vi "Weather Parse Test.vi"() -> ()   [LabVIEW 2020, in "CDM-Config.lvlib"] (continued)
                 ],\n                    \"WMOidentifier\": [\n                        \"FZAK51 PAFC 021149\"\n                    ],\n                    \"NWSheadline\": [\n                        \"SMALL CRAFT ADVISORY THROUGH WEDNESDAY\"\n                    ],\n                    \"BLOCKCHANNEL\": [\n                        \"EAS\",\n                        \"NWEM\",\n                        \"CMAS\"\n                    ],\n                    \"VTEC\": [\n                        \"/O.NEW.PAFC.SC.Y.9557.251202T1100Z-251204T0200Z/\"\n                    ],\n                    \"eventEndingTime\": [\n                        \"2025-12-03T17:00:00-09:00\"\n                    ]\n                },\n                \"scope\": \"Public\",\n                \"code\": \"IPAWSv1.0\",\n                \"language\": \"en-US\",\n                \"web\": \"http://www.weather.gov\",\n                \"eventCode\": {\n                    \"SAME\": [\n                        \"NWS\"\n                    ],\n                    \"NationalWeatherService\": [\n                        \"SCY\"\n                    ]\n                }\n            }\n        },\n        {\n            \"id\": \"https://api.weather.gov/alerts/urn:oid:2.49.0.1.840.0.7a1ebf60c096e67f68143934abaf6f7cf8a57038.003.1\",\n            \"type\": \"Feature\",\n            \"geometry\": null,\n            \"properties\": {\n                \"@id\": \"https://api.weather.gov/alerts/urn:oid:2.49.0.1.840.0.7a1ebf60c096e67f68143934abaf6f7cf8a57038.003.1\",\n                \"@type\": \"wx:Alert\",\n                \"id\": \"urn:oid:2.49.0.1.840.0.7a1ebf60c096e67f68143934abaf6f7cf8a57038.003.1\",\n                \"areaDesc\": \"Gravel Point to Cape Cleare out to 15 NM\",\n                \"geocode\": {\n                    \"SAME\": [\n                        \"058711\"\n                    ],\n                    \"UGC\": [\n                        \"PKZ711\"\n                    ]\n                },\n                \"affectedZones\": [\n                    \"https://api.weather.gov/zones/forecast/PKZ711\"\n                ],\n                \"references\": [],\n                \"sent\": \"2025-12-02T02:49:00-09:00\",\n                \"effective\": \"2025-12-02T02:49:00-09:00\",\n                \"onset\": \"2025-12-02T02:00:00-09:00\",\n                \"expires\": \"2025-12-02T15:45:00-09:00\",\n                \"ends\": \"2025-12-03T17:00:00-09:00\",\n                \"status\": \"Actual\",\n                \"messageType\": \"Alert\",\n                \"category\": \"Met\",\n                \"severity\": \"Minor\",\n                \"certainty\": \"Likely\",\n                \"urgency\": \"Expected\",\n                \"event\": \"Small Craft Advisory\",\n                \"sender\": \"w-nws.webmaster@noaa.gov\",\n                \"senderName\": \"NWS Anchorage AK\",\n                \"headline\": \"Small Craft Advisory issued December 2 at 2:49AM AKST until December 3 at 5:00PM AKST by NWS Anchorage AK\",\n                \"description\": \"Coastal Waters Forecast for the Northern Gulf of Alaska Coast\\nup to 100 nm out including Kodiak Island and Cook Inlet.\\n\\nWind forecasts reflect the predominant speed and direction\\nexpected. Sea forecasts represent an average of the highest\\none-third of the combined wind wave and swell height.\\n\\n.TODAY...SE wind 25 kt. Seas 8 ft. Rain.\\n.TONIGHT...SE wind 25 kt. Seas 9 ft.\\n.WED...E wind 15 kt. Seas 9 ft.\\n.WED NIGHT...Variable wind 10 kt. Seas 8 ft.\\n.THU...Variable wind 10 kt. Seas 7 ft.\\n.FRI...Variable wind 10 kt. Seas 5 ft.\\n.SAT...SE wind 20 kt. Seas 9 ft.\",\n                \"instruction\": null,\n                \"response\": \"Avoid\",\n                \"parameters\": {\n                    \"AWIPSidentifier\": [\n                        \"CWFAER\"\n                    ],\n                    \"WMOidentifier\": [\n                        \"FZAK51 PAFC 021149\"\n                    ],\n                    \"NWSheadline\": [\n                        \"SMALL CRAFT ADVISORY THROUGH WEDNESDAY\"\n                    ],\n                    \"BLOCKCHANNEL\": [\n                        \"EAS\",\n                        \"NWEM\",\n                        \"CMAS\"\n                    ],\n                    \"VTEC\": [\n                        \"/O.NEW.PAFC.SC.Y.9558.251202T1100Z-251204T0200Z/\"\n                    ],\n                    \"eventEndingTime\": [\n                        \"2025-12-03T17:00:00-09:00\"\n                    ]\n                },\n                \"scope\": \"Public\",\n                \"code\": \"IPAWSv1.0\",\n                \"language\": \"en-US\",\n                \"web\": \"http://www.weather.gov\",\n                \"eventCode\": {\n                    \"SAME\": [\n                        \"NWS\"\n                    ],\n                    \"NationalWeatherService\": [\n                        \"SCY\"\n                    ]\n                }\n            }\n        },\n        {\n            \"id\": \"https://api.weather.gov/alerts/urn:oid:2.49.0.1.840.0.7a1ebf60c096e67f68143934abaf6f7cf8a57038.017.1\",\n            \"type\": \"Feature\",\n            \"geometry\": null,\n            \"properties\": {\n                \"@id\": \"https://api.weather.gov/alerts/urn:oid:2.49.0.1.840.0.7a1ebf60c096e67f68143934abaf6f7cf8a57038.017.1\",\n                \"@type\": \"wx:Alert\",\n                \"id\": \"urn:oid:2.49.0.1.840.0.7a1ebf60c096e67f68143934abaf6f7cf8a57038.017.1\",\n                \"areaDesc\": \"Gore Point to Marmot Island from 15 to 80 NM\",\n                \"geocode\": {\n                    \"SAME\": [\n                        \"058733\"\n                    ],\n                    \"UGC\": [\n                        \"PKZ733\"\n                    ]\n                },\n                \"affectedZones\": [\n                    \"https://api.weather.gov/zones/forecast/PKZ733\"\n                ],\n                \"references\": [],\n                \"sent\": \"2025-12-02T02:49:00-09:00\",\n                \"effective\": \"2025-12-02T02:49:00-09:00\",\n                \"onset\": \"2025-12-02T02:00:00-09:00\",\n                \"expires\": \"2025-12-02T15:45:00-09:00\",\n                \"ends\": \"2025-12-03T17:00:00-09:00\",\n                \"status\": \"Actual\",\n                \"messageType\": \"Alert\",\n                \"category\": \"Met\",\n                \"severity\": \"Minor\",\n                \"certainty\": \"Likely\",\n                \"urgency\": \"Expected\",\n                \"event\": \"Small Craft Advisory\",\n                \"sender\": \"w-nws.webmaster@noaa.gov\",\n                \"senderName\": \"NWS Anchorage AK\",\n                \"headline\": \"Small Craft Advisory issued December 2 at 2:49AM AKST until December 3 at 5:00PM AKST by NWS Anchorage AK\",\n                \"description\": \"Coastal Waters Forecast for the Northern Gulf of Alaska Coast\\nup to 100 nm out including Kodiak Island and Cook Inlet.\\n\\nWind forecasts reflect the predominant speed and direction\\nexpected. Sea forecasts represent an average of the highest\\none-third of the combined wind wave and swell height.\\n\\n.TODAY...SE wind 30 kt becoming S 15 kt in the afternoon. Seas\\n11 ft.\\n.TONIGHT...Variable wind 10 kt. Seas 11 ft.\\n.WED...Variable wind 10 kt. Seas 10 ft.\\n.WED NIGHT...SW wind 15 kt. Seas 9 ft.\\n.THU...Variable wind 10 kt. Seas 8 ft.\\n.FRI...SW wind 15 kt. Seas 9 ft.\\n.SAT...Variable wind 10 kt. Seas 9 ft.\",\n                \"instruction\": null,\n                \"response\": \"Avoid\",\n                \"parameters\": {\n                    \"AWIPSidentifier\": [\n                        \"CWFAER\"\n                    ],\n                    \"WMOidentifier\": [\n                        \"FZAK51 PAFC 021149\"\n                    ],\n                    \"NWSheadline\": [\n                        \"SMALL CRAFT ADVISORY THROUGH WEDNESDAY\"\n                    ],\n                    \"BLOCKCHANNEL\": [\n                        \"EAS\",\n                        \"NWEM\",\n                        \"CMAS\"\n                    ],\n                    \"VTEC\": [\n                        \"/O.NEW.PAFC.SC.Y.9565.251202T1100Z-251204T0200Z/\"\n                    ],\n                    \"eventEndingTime\": [\n                        \"2025-12-03T17:00:00-09:00\"\n                    ]\n                },\n                \"scope\": \"Public\",\n                \"code\": \"IPAWSv1.0\",\n                \"language\": \"en-US\",\n                \"web\": \"http://www.weather.gov\",\n                \"eventCode\": {\n                    \"SAME\": [\n                        \"NWS\"\n                    ],\n                    \"NationalWeatherService\": [\n                        \"SCY\"\n                    ]\n                }\n            }\n        },\n        {\n            \"id\": \"https://api.weather.gov/alerts/urn:oid:2.49.0.1.840.0.7a1ebf60c096e67f68143934abaf6f7cf8a57038.004.1\",\n            \"type\": \"Feature\",\n            \"geometry\": null,\n            \"properties\": {\n                \"@id\": \"https://api.weather.gov/alerts/urn:oid:2.49.0.1.840.0.7a1ebf60c096e67f68143934abaf6f7cf8a57038.004.1\",\n                \"@type\": \"wx:Alert\",\n                \"id\": \"urn:oid:2.49.0.1.840.0.7a1ebf60c096e67f68143934abaf6f7cf8a57038.004.1\",\n                \"areaDesc\": \"Cape Suckling to Cape Cleare from 15 to 75 NM\",\n                \"geocode\": {\n                    \"SAME\": [\n                        \"058712\"\n                    ],\n                    \"UGC\": [\n                        \"PKZ712\"\n                    ]\n                },\n                \"affectedZones\": [\n                    \"https://api.weather.gov/zones/forecast/PKZ712\"\n                ],\n                \"references\": [],\n                \"sent\": \"2025-12-02T02:49:00-09:00\",\n                \"effective\": \"2025-12-02T02:49:00-09:00\",\n                \"onset\": \"2025-12-02T02:00:00-09:00\",\n                \"expires\": \"2025-12-02T15:45:00-09:00\",\n                \"ends\": \"2025-12-03T17:00:00-09:00\",\n                \"status\": \"Actual\",\n                \"messageType\": \"Alert\",\n                \"category\": \"Met\",\n                \"severity\": \"Minor\",\n                \"certainty\": \"Likely\",\n                \"urgency\": \"Expected\",\n                \"event\": \"Small Craft Advisory\",\n                \"sender\": \"w-nws.webmaster@noaa.gov\",\n                \"senderName\": \"NWS Anchorage AK\",\n                \"headline\": \"Small Craft Advisory issued December 2 at 2:49AM AKST until December 3 at 5:00PM AKST by NWS Anchorage AK\",\n                \"description\": \"Coastal Waters Forecast for the Northern Gulf of Alaska Coast\\nup to 100 nm out including Kodiak Island and Cook Inlet.\\n\\nWind forecasts reflect the predominant speed and direction\\nexpected. Sea forecasts represent an average of the highest\\none-third of the combined wind wave and swell height.\\n\\n.TODAY...SE wind 25 kt. Seas 10 ft. Rain.\\n.TONIGHT...SE wind 20 kt. Seas 10 ft.\\n.WED...Variable wind 10 kt. Seas 11 ft.\\n.WED NIGHT...W wind 15 kt. Seas 10 ft.\\n.THU...Variable wind 10 kt. Seas 8 ft.\\n.FRI...SE wind 15 kt. Seas 6 ft.\\n.SAT...SE wind 20 kt. Seas 9 ft.\",\n                \"instruction\": null,\n                \"response\": \"Avoid\",\n                \"parameters\": {\n                    \"AWIPSidentifier\": [\n                        \"CWFAER\"\n                    ],\n                    \"WMOidentifier\": [\n                        \"FZAK51 PAFC 021149\"\n                    ],\n                    \"NWSheadline\": [\n                        \"SMALL CRAFT ADVISORY THROUGH WEDNESDAY\"\n                    ],\n                    \"BLOCKCHANNEL\": [\n                        \"EAS\",\n                        \"NWEM\",\n                        \"CMAS\"\n                    ],\n                    \"VTEC\": [\n                        \"/O.NEW.PAFC.SC.Y.9559.251202T1100Z-251204T0200Z/\"\n                    ],\n                    \"eventEndingTime\": [\n                        \"2025-12-03T17:00:00-09:00\"\n                    ]\n                },\n                \"scope\": \"Public\",\n                \"code\": \"IPAWSv1.0\",\n                \"language\": \"en-US\",\n                \"web\": \"http://www.weather.gov\",\n                \"eventCode\": {\n                    \"SAME\": [\n                        \"NWS\"\n                    ],\n                    \"NationalWeatherService\": [\n                        \"SCY\"\n                    ]\n                }\n            }\n        },\n        {\n            \"id\": \"https://api.weather.gov/alerts/urn:oid:2.49.0.1.840.0.7a1ebf60c096e67f68143934abaf6f7cf8a57038.019.1\",\n            \"type\": \"Feature\",\n            \"geometry\": null,\n            \"properties\": {\n                \"@id\": \"https://api.weather.gov/alerts/urn:oid:2.49.0.1.840.0.7a1ebf60c096e67f68143934abaf6f7cf8a57038.019.1\",\n                \"@type\": \"wx:Alert\",\n                \"id\": \"urn:oid:2.49.0.1.840.0.7a1ebf60c096e67f68143934abaf6f7cf8a57038.019.1\",\n                \"areaDesc\": \"Marmot Island To Sitkinak from 15 to 85 NM\",\n                \"geocode\": {\n                    \"SAME\": [\n                        \"058734\"\n                    ],\n                    \"UGC\": [\n                        \"PKZ734\"\n                    ]\n                },\n                \"affectedZones\": [\n                    \"https://api.weather.gov/zones/forecast/PKZ734\"\n                ],\n                \"references\": [],\n                \"sent\": \"2025-12-02T02:49:00-09:00\",\n                \"effective\": \"2025-12-02T02:49:00-09:00\",\n                \"onset\": \"2025-12-02T02:00:00-09:00\",\n                \"expires\": \"2025-12-02T15:45:00-09:00\",\n                \"ends\": \"2025-12-03T17:00:00-09:00\",\n                \"status\": \"Actual\",\n                \"messageType\": \"Alert\",\n                \"category\": \"Met\",\n                \"severity\": \"Minor\",\n                \"certainty\": \"Likely\",\n                \"urgency\": \"Expected\",\n                \"event\": \"Small Craft Advisory\",\n                \"sender\": \"w-nws.webmaster@noaa.gov\",\n                \"senderName\": \"NWS Anchorage AK\",\n                \"headline\": \"Small Craft Advisory issued December 2 at 2:49AM AKST until December 3 at 5:00PM AKST by NWS Anchorage AK\",\n                \"description\": \"Coastal Waters Forecast for the Northern Gulf of Alaska Coast\\nup to 100 nm out including Kodiak Island and Cook Inlet.\\n\\nWind forecasts reflect the predominant speed and direction\\nexpected. Sea forecasts represent an average of the highest\\none-third of the combined wind wave and swell height.\\n\\n.TODAY...S wind 25 kt. Seas 16 ft.\\n.TONIGHT...SE wind 20 kt. Seas 15 ft.\\n.WED...S wind 20 kt. Seas 13 ft.\\n.WED NIGHT...S wind 15 kt. Seas 10 ft.\\n.THU...E wind 20 kt. Seas 9 ft.\\n.FRI...W wind 15 kt. Seas 9 ft.\\n.SAT...NW wind 25 kt. Seas 10 ft.\",\n                \"instruction\": null,\n                \"response\": \"Avoid\",\n                \"parameters\": {\n                    \"AWIPSidentifier\": [\n                        \"CWFAER\"\n                    ],\n                    \"WMOidentifier\": [\n                        \"FZAK51 PAFC 021149\"\n                    ],\n                    \"NWSheadline\": [\n                        \"SMALL CRAFT ADVISORY THROUGH WEDNESDAY\"\n                    ],\n                    \"BLOCKCHANNEL\": [\n                        \"EAS\",\n                        \"NWEM\",\n                        \"CMAS\"\n                    ],\n                    \"VTEC\": [\n                        \"/O.NEW.PAFC.SC.Y.9567.251202T1100Z-251204T0200Z/\"\n                    ],\n                    \"eventEndingTime\": [\n                        \"2025-12-03T17:00:00-09:00\"\n                    ]\n                },\n                \"scope\": \"Public\",\n                \"code\": \"IPAWSv1.0\",\n                \"language\": \"en-US\",\n                \"web\": \"http://www.weather.gov\",\n                \"eventCode\": {\n                    \"SAME\": [\n                        \"NWS\"\n                    ],\n                    \"NationalWeatherService\": [\n                        \"SCY\"\n                    ]\n                }\n            }\n        },\n        {\n            \"id\": \"https://api.weather.gov/alerts/urn:oid:2.49.0.1.840.0.8d8456a64db8f93a127de0b73ddc98c3f937e864.024.1\",\n            \"type\": \"Feature\",\n            \"geometry\": null,\n            \"properties\": {\n                \"@id\": \"https://api.weather.gov/alerts/urn:oid:2.49.0.1.840.0.8d8456a64db8f93a127de0b73ddc98c3f937e864.024.1\",\n                \"@type\": \"wx:Alert\",\n                \"id\": \"urn:oid:2.49.0.1.840.0.8d8456a64db8f93a127de0b73ddc98c3f937e864.024.1\",\n                \"areaDesc\": \"Seguam to Adak Pacific Side from 15 to 75 NM\",\n                \"geocode\": {\n                    \"SAME\": [\n                        \"058783\"\n                    ],\n                    \"UGC\": [\n                        \"PKZ783\"\n                    ]\n                },\n                \"affectedZones\": [\n                    \"https://api.weather.gov/zones/forecast/PKZ783\"\n                ],\n                \"references\": [],\n                \"sent\": \"2025-12-02T02:49:00-09:00\",\n                \"effective\": \"2025-12-02T02:49:00-09:00\",\n                \"onset\": \"2025-12-02T02:00:00-09:00\",\n                \"expires\": \"2025-12-02T15:45:00-09:00\",\n                \"ends\": \"2025-12-03T17:00:00-09:00\",\n                \"status\": \"Actual\",\n                \"messageType\": \"Alert\",\n                \"category\": \"Met\",\n                \"severity\": \"Moderate\",\n                \"certainty\": \"Likely\",\n                \"urgency\": \"Expected\",\n                \"event\": \"Gale Warning\",\n                \"sender\": \"w-nws.webmaster@noaa.gov\",\n                \"senderName\": \"NWS Anchorage AK\",\n                \"headline\": \"Gale Warning issued December 2 at 2:49AM AKST until December 3 at 5:00PM AKST by NWS Anchorage AK\",\n                \"description\": \"Coastal Waters Forecast for Southwest Alaska+Bristol Bay+The\\nAlaska Peninsula Waters and the Aleutian Islands up to 100 nm out.\\n\\nWind forecasts reflect the predominant speed and direction\\nexpected. Sea forecasts represent an average of the highest\\none-third of the combined wind wave and swell height.\\n\\n.TODAY...N wind 40 kt. Seas 18 ft. Rain with snow.\\n.TONIGHT...NW wind 45 kt. Seas 20 ft.\\n.WED...N wind 35 kt. Seas 16 ft.\\n.WED NIGHT...N wind 30 kt. Seas 14 ft.\\n.THU...N wind 30 kt. Seas 11 ft.\\n.FRI...W wind 20 kt. Seas 15 ft.\\n.SAT...NE wind 15 kt. Seas 13 ft.\",\n                \"instruction\": null,\n                \"response\": \"Avoid\",\n                \"parameters\": {\n                    \"AWIPSidentifier\": [\n                        \"CWFALU\"\n                    ],\n                    \"WMOidentifier\": [\n                        \"FZAK52 PAFC 021149\"\n                    ],\n                    \"NWSheadline\": [\n                        \"GALE WARNING THROUGH WEDNESDAY\"\n                    ],\n                    \"BLOCKCHANNEL\": [\n                        \"EAS\",\n                        \"NWEM\",\n                        \"CMAS\"\n                    ],\n                    \"VTEC\": [\n                        \"/O.NEW.PAFC.GL.W.3161.251202T1100Z-251204T0200Z/\"\n                    ],\n                    \"eventEndingTime\": [\n                        \"2025-12-03T17:00:00-09:00\"\n                    ]\n                },\n                \"scope\": \"Public\",\n                \"code\": \"IPAWSv1.0\",\n                \"language\": \"en-US\",\n                \"web\": \"http://www.weather.gov\",\n                \"eventCode\": {\n                    \"SAME\": [\n                        \"NWS\"\n                    ],\n                    \"NationalWeatherService\": [\n                        \"GLW\"\n                    ]\n                }\n            }\n        },\n        {\n            \"id\": \"https://api.weather.gov/alerts/urn:oid:2.49.0.1.840.0.8d8456a64db8f93a127de0b73ddc98c3f937e864.018.1\",\n            \"type\": \"Feature\",\n            \"geometry\": null,\n            \"properties\": {\n                \"@id\": \"https://api.weather.gov/alerts/urn:oid:2.49.0.1.840.0.8d8456a64db8f93a127de0b73ddc98c3f937e864.018.1\",\n                \"@type\": \"wx:Alert\",\n                \"id\": \"urn:oid:2.49.0.1.840.0.8d8456a64db8f93a127de0b73ddc98c3f937e864.018.1\",\n                \"areaDesc\": \"Nikolski to Seguam Bering Side from 15 to 85 NM\",\n                \"geocode\": {\n                    \"SAME\": [\n                        \"058776\"\n                    ],\n                    \"UGC\": [\n                        \"PKZ776\"\n                    ]\n                },\n                \"affectedZones\": [\n                    \"https://api.weather.gov/zones/forecast/PKZ776\"\n                ],\n                \"references\": [],\n                \"sent\": \"2025-12-02T02:49:00-09:00\",\n                \"effective\": \"2025-12-02T02:49:00-09:00\",\n                \"onset\": \"2025-12-02T02:00:00-09:00\",\n                \"expires\": \"2025-12-02T15:45:00-09:00\",\n                \"ends\": \"2025-12-03T17:00:00-09:00\",\n                \"status\": \"Actual\",\n                \"messageType\": \"Alert\",\n                \"category\": \"Met\",\n                \"severity\": \"Moderate\",\n                \"certainty\": \"Likely\",\n                \"urgency\": \"Expected\",\n                \"event\": \"Gale Warning\",\n                \"sender\": \"w-nws.webmaster@noaa.gov\",\n                \"senderName\": \"NWS Anchorage AK\",\n                \"headline\": \"Gale Warning issued December 2 at 2:49AM AKST until December 3 at 5:00PM AKST by NWS Anchorage AK\",\n                \"description\": \"Coastal Waters Forecast for Southwest Alaska+Bristol Bay+The\\nAlaska Peninsula Waters and the Aleutian Islands up to 100 nm out.\\n\\nWind forecasts reflect the predominant speed and direction\\nexpected. Sea forecasts represent an average of the highest\\none-third of the combined wind wave and swell height.\\n\\n.TODAY...N wind 45 kt. Seas 29 ft. Rain.\\n.TONIGHT...NE wind 45 kt becoming N 35 kt after midnight. Seas\\n30 ft. Rain.\\n.WED...N wind 35 kt. Seas 23 ft.\\n.WED NIGHT...N wind 30 kt. Seas 21 ft.\\n.THU...NE wind 30 kt. Seas 16 ft.\\n.FRI...NE wind 15 kt. Seas 9 ft.\\n.SAT...N wind 20 kt. Seas 10 ft.\",\n                \"instruction\": null,\n                \"response\": \"Avoid\",\n                \"parameters\": {\n                    \"AWIPSidentifier\": [\n                        \"CWFALU\"\n                    ],\n                    \"WMOidentifier\": [\n                        \"FZAK52 PAFC 021149\"\n                    ],\n                    \"NWSheadline\": [\n                        \"GALE WARNING THROUGH WEDNESDAY\"\n                    ],\n                    \"BLOCKCHANNEL\": [\n                        \"EAS\",\n                        \"NWEM\",\n                        \"CMAS\"\n                    ],\n                    \"VTEC\": [\n                        \"/O.NEW.PAFC.GL.W.3155.251202T1100Z-251204T0200Z/\"\n                    ],\n                    \"eventEndingTime\": [\n                        \"2025-12-03T17:00:00-09:00\"\n                    ]\n                },\n                \"scope\": \"Public\",\n                \"code\": \"IPAWSv1.0\",\n                \"language\": \"en-US\",\n                \"web\": \"http://www.weather.gov\",\n                \"eventCode\": {\n                    \"SAME\": [\n                        \"NWS\"\n                    ],\n                    \"NationalWeatherService\": [\n                        \"GLW\"\n                    ]\n                }\n            }\n        },\n        {\n            \"id\": \"https://api.weather.gov/alerts/urn:oid:2.49.0.1.840.0.8d8456a64db8f93a127de0b73ddc98c3f937e864.022.1\",\n            \"type\": \"Feature\",\n            \"geometry\": null,\n            \"properties\": {\n                \"@id\": \"https://api.weather.gov/alerts/urn:oid:2.49.0.1.840.0.8d8456a64db8f93a127de0b73ddc98c3f937e864.022.1\",\n                \"@type\": \"wx:Alert\",\n                \"id\": \"urn:oid:2.49.0.1.840.0.8d8456a64db8f93a127de0b73ddc98c3f937e864.022.1\",\n                \"areaDesc\": \"Seguam to Adak Bering Side from 15 to 85 NM\",\n                \"geocode\": {\n                    \"SAME\": [\n                        \"058781\"\n                    ],\n                    \"UGC\": [\n                        \"PKZ781\"\n                    ]\n                },\n                \"affectedZones\": [\n                    \"https://api.weather.gov/zones/forecast/PKZ781\"\n                ],\n                \"references\": [],\n                \"sent\": \"2025-12-02T02:49:00-09:00\",\n                \"effective\": \"2025-12-02T02:49:00-09:00\",\n                \"onset\": \"2025-12-02T02:00:00-09:00\",\n                \"expires\": \"2025-12-02T15:45:00-09:00\",\n                \"ends\": \"2025-12-03T17:00:00-09:00\",\n                \"status\": \"Actual\",\n                \"messageType\": \"Alert\",\n                \"category\": \"Met\",\n                \"severity\": \"Moderate\",\n                \"certainty\": \"Likely\",\n                \"urgency\": \"Expected\",\n                \"event\": \"Gale Warning\",\n                \"sender\": \"w-nws.webmaster@noaa.gov\",\n                \"senderName\": \"NWS Anchorage AK\",\n                \"headline\": \"Gale Warning issued December 2 at 2:49AM AKST until December 3 at 5:00PM AKST by NWS Anchorage AK\",\n                \"description\": \"Coastal Waters Forecast for Southwest Alaska+Bristol Bay+The\\nAlaska Peninsula Waters and the Aleutian Islands up to 100 nm out.\\n\\nWind forecasts reflect the predominant speed and direction\\nexpected. Sea forecasts represent an average of the highest\\none-third of the combined wind wave and swell height.\\n\\n.TODAY...N wind 45 kt. Seas 31 ft. Rain with snow.\\n.TONIGHT...N wind 45 kt. Seas 31 ft. Rain and snow.\\n.WED...N wind 40 kt. Seas 28 ft.\\n.WED NIGHT...N wind 30 kt. Seas 22 ft.\\n.THU...NE wind 30 kt. Seas 16 ft.\\n.FRI THROUGH SAT...NE wind 15 kt. Seas 9 ft.\",\n                \"instruction\": null,\n                \"response\": \"Avoid\",\n                \"parameters\": {\n                    \"AWIPSidentifier\": [\n                        \"CWFALU\"\n                    ],\n                    \"WMOidentifier\": [\n                        \"FZAK52 PAFC 021149\"\n                    ],\n                    \"NWSheadline\": [\n                        \"GALE WARNING THROUGH WEDNESDAY\"\n                    ],\n                    \"BLOCKCHANNEL\": [\n                        \"EAS\",\n                        \"NWEM\",\n                        \"CMAS\"\n                    ],\n                    \"VTEC\": [\n                        \"/O.NEW.PAFC.GL.W.3159.251202T1100Z-251204T0200Z/\"\n                    ],\n                    \"eventEndingTime\": [\n                        \"2025-12-03T17:00:00-09:00\"\n                    ]\n                },\n                \"scope\": \"Public\",\n                \"code\": \"IPAWSv1.0\",\n                \"language\": \"en-US\",\n                \"web\": \"http://www.weather.gov\",\n                \"eventCode\": {\n                    \"SAME\": [\n                        \"NWS\"\n                    ],\n                    \"NationalWeatherService\": [\n                        \"GLW\"\n                    ]\n                }\n            }\n        },\n        {\n            \"id\": \"https://api.weather.gov/alerts/urn:oid:2.49.0.1.840.0.8d8456a64db8f93a127de0b73ddc98c3f937e864.023.1\",\n            \"type\": \"Feature\",\n            \"geometry\": null,\n            \"properties\": {\n                \"@id\": \"https://api.weather.gov/alerts/urn:oid:2.49.0.1.840.0.8d8456a64db8f93a127de0b73ddc98c3f937e864.023.1\",\n                \"@type\": \"wx:Alert\",\n                \"id\": \"urn:oid:2.49.0.1.840.0.8d8456a64db8f93a127de0b73ddc98c3f937e864.023.1\",\n                \"areaDesc\": \"Seguam to Adak Pacific Side out to 15 NM\",\n                \"geocode\": {\n                    \"SAME\": [\n                        \"058782\"\n                    ],\n                    \"UGC\": [\n                        \"PKZ782\"\n                    ]\n                },\n                \"affectedZones\": [\n                    \"https://api.weather.gov/zones/forecast/PKZ782\"\n                ],\n                \"references\": [],\n                \"sent\": \"2025-12-02T02:49:00-09:00\",\n                \"effective\": \"2025-12-02T02:49:00-09:00\",\n                \"onset\": \"2025-12-02T02:00:00-09:00\",\n                \"expires\": \"2025-12-02T15:45:00-09:00\",\n                \"ends\": \"2025-12-03T17:00:00-09:00\",\n                \"status\": \"Actual\",\n                \"messageType\": \"Alert\",\n                \"category\": \"Met\",\n                \"severity\": \"Moderate\",\n                \"certainty\": \"Likely\",\n                \"urgency\": \"Expected\",\n                \"event\": \"Gale Warning\",\n                \"sender\": \"w-nws.webmaster@noaa.gov\",\n                \"senderName\": \"NWS Anchorage AK\",\n                \"headline\": \"Gale Warning issued December 2 at 2:49AM AKST until December 3 at 5:00PM AKST by NWS Anchorage AK\",\n                \"description\": \"Coastal Waters Forecast for Southwest Alaska+Bristol Bay+The\\nAlaska Peninsula Waters and the Aleutian Islands up to 100 nm out.\\n\\nWind forecasts reflect the predominant speed and direction\\nexpected. Sea forecasts represent an average of the highest\\none-third of the combined wind wave and swell height.\\n\\n.TODAY...N wind 40 kt. Seas 15 ft. Rain and snow.\\n.TONIGHT...N wind 45 kt. Seas 15 ft. Rain and snow.\\n.WED...N wind 35 kt. Seas 14 ft.\\n.WED NIGHT...N wind 30 kt. Seas 12 ft.\\n.THU...N wind 30 kt. Seas 9 ft.\\n.FRI...NW wind 15 kt. Seas 12 ft.\\n.SAT...NE wind 15 kt. Seas 12 ft.\",\n                \"instruction\": null,\n                \"response\": \"Avoid\",\n                \"parameters\": {\n                    \"AWIPSidentifier\": [\n                        \"CWFALU\"\n                    ],\n                    \"WMOidentifier\": [\n                        \"FZAK52 PAFC 021149\"\n                    ],\n                    \"NWSheadline\": [\n                        \"GALE WARNING THROUGH WEDNESDAY\"\n                    ],\n                    \"BLOCKCHANNEL\": [\n                        \"EAS\",\n                        \"NWEM\",\n                        \"CMAS\"\n                    ],\n                    \"VTEC\": [\n                        \"/O.NEW.PAFC.GL.W.3160.251202T1100Z-251204T0200Z/\"\n                    ],\n                    \"eventEndingTime\": [\n                        \"2025-12-03T17:00:00-09:00\"\n                    ]\n                },\n                \"scope\": \"Public\",\n                \"code\": \"IPAWSv1.0\",\n                \"language\": \"en-US\",\n                \"web\": \"http://www.weather.gov\",\n                \"eventCode\": {\n                    \"SAME\": [\n                        \"NWS\"\n                    ],\n                    \"NationalWeatherService\": [\n                        \"GLW\"\n                    ]\n                }\n            }\n        },\n        {\n            \"id\": \"https://api.weather.gov/alerts/urn:oid:2.49.0.1.840.0.8d8456a64db8f93a127de0b73ddc98c3f937e864.003.1\",\n            \"type\": \"Feature\",\n            \"geometry\": null,\n            \"properties\": {\n                \"@id\": \"https://api.weather.gov/alerts/urn:oid:2.49.0.1.840.0.8d8456a64db8f93a127de0b73ddc98c3f937e864.003.1\",\n                \"@type\": \"wx:Alert\",\n                \"id\": \"urn:oid:2.49.0.1.840.0.8d8456a64db8f93a127de0b73ddc98c3f937e864.003.1\",\n                \"areaDesc\": \"Sitkinak to Castle Cape from 15 to 100 NM\",\n                \"geocode\": {\n                    \"SAME\": [\n                        \"058751\"\n                    ],\n                    \"UGC\": [\n                        \"PKZ751\"\n                    ]\n                },\n                \"affectedZones\": [\n                    \"https://api.weather.gov/zones/forecast/PKZ751\"\n                ],\n                \"references\": [],\n                \"sent\": \"2025-12-02T02:49:00-09:00\",\n                \"effective\": \"2025-12-02T02:49:00-09:00\",\n                \"onset\": \"2025-12-02T02:00:00-09:00\",\n                \"expires\": \"2025-12-02T15:45:00-09:00\",\n                \"ends\": \"2025-12-03T17:00:00-09:00\",\n                \"status\": \"Actual\",\n                \"messageType\": \"Alert\",\n                \"category\": \"Met\",\n                \"severity\": \"Minor\",\n                \"certainty\": \"Likely\",\n                \"urgency\": \"Expected\",\n                \"event\": \"Small Craft Advisory\",\n                \"sender\": \"w-nws.webmaster@noaa.gov\",\n                \"senderName\": \"NWS Anchorage AK\",\n                \"headline\": \"Small Craft Advisory issued December 2 at 2:49AM AKST until December 3 at 5:00PM AKST by NWS Anchorage AK\",\n                \"description\": \"Coastal Waters Forecast for Southwest Alaska+Bristol Bay+The\\nAlaska Peninsula Waters and the Aleutian Islands up to 100 nm out.\\n\\nWind forecasts reflect the predominant speed and direction\\nexpected. Sea forecasts represent an average of the highest\\none-third of the combined wind wave and swell height.\\n\\n.TODAY...S wind 30 kt. Seas 21 ft.\\n.TONIGHT...SE wind 25 kt. Seas 18 ft.\\n.WED...S wind 20 kt. Seas 14 ft.\\n.WED NIGHT...SE wind 20 kt. Seas 13 ft.\\n.THU...E wind 20 kt. Seas 11 ft.\\n.FRI...W wind 15 kt. Seas 7 ft.\\n.SAT...NW wind 25 kt. Seas 9 ft.\",\n                \"instruction\": null,\n                \"response\": \"Avoid\",\n                \"parameters\": {\n                    \"AWIPSidentifier\": [\n                        \"CWFALU\"\n                    ],\n                    \"WMOidentifier\": [\n                        \"FZAK52 PAFC 021149\"\n                    ],\n                    \"NWSheadline\": [\n                        \"SMALL CRAFT ADVISORY THROUGH WEDNESDAY\"\n                    ],\n                    \"BLOCKCHANNEL\": [\n                        \"EAS\",\n                        \"NWEM\",\n                        \"CMAS\"\n                    ],\n                    \"VTEC\": [\n                        \"/O.NEW.PAFC.SC.Y.3140.251202T1100Z-251204T0200Z/\"\n                    ],\n                    \"eventEndingTime\": [\n                        \"2025-12-03T17:00:00-09:00\"\n                    ]\n                },\n                \"scope\": \"Public\",\n                \"code\": \"IPAWSv1.0\",\n                \"language\": \"en-US\",\n                \"web\": \"http://www.weather.gov\",\n                \"eventCode\": {\n                    \"SAME\": [\n                        \"NWS\"\n                    ],\n                    \"NationalWeatherService\": [\n                        \"SCY\"\n                    ]\n                }\n            }\n        },\n        {\n            \"id\": \"https://api.weather.gov/alerts/urn:oid:2.49.0.1.840.0.8d8456a64db8f93a127de0b73ddc98c3f937e864.002.1\",\n            \"type\": \"Feature\",\n            \"geometry\": null,\n            \"properties\": {\n                \"@id\": \"https://api.weather.gov/alerts/urn:oid:2.49.0.1.840.0.8d8456a64db8f93a127de0b73ddc98c3f937e864.002.1\",\n                \"@type\": \"wx:Alert\",\n                \"id\": \"urn:oid:2.49.0.1.840.0.8d8456a64db8f93a127de0b73ddc98c3f937e864.002.1\",\n                \"areaDesc\": \"Sitkinak to Castle Cape out to 15 NM\",\n                \"geocode\": {\n                    \"SAME\": [\n                        \"058750\"\n                    ],\n                    \"UGC\": [\n                        \"PKZ750\"\n                    ]\n                },\n                \"affectedZones\": [\n                    \"https://api.weather.gov/zones/forecast/PKZ750\"\n                ],\n                \"references\": [],\n                \"sent\": \"2025-12-02T02:49:00-09:00\",\n                \"effective\": \"2025-12-02T02:49:00-09:00\",\n                \"onset\": \"2025-12-02T02:00:00-09:00\",\n                \"expires\": \"2025-12-02T15:45:00-09:00\",\n                \"ends\": \"2025-12-03T17:00:00-09:00\",\n                \"status\": \"Actual\",\n                \"messageType\": \"Alert\",\n                \"category\": \"Met\",\n                \"severity\": \"Minor\",\n                \"certainty\": \"Likely\",\n                \"urgency\": \"Expected\",\n                \"event\": \"Small Craft Advisory\",\n                \"sender\": \"w-nws.webmaster@noaa.gov\",\n                \"senderName\": \"NWS Anchorage AK\",\n                \"headline\": \"Small Craft Advisory issued December 2 at 2:49AM AKST until December 3 at 5:00PM AKST by NWS Anchorage AK\",\n                \"description\": \"Coastal Waters Forecast for Southwest Alaska+Bristol Bay+The\\nAlaska Peninsula Waters and the Aleutian Islands up to 100 nm out.\\n\\nWind forecasts reflect the predominant speed and direction\\nexpected. Sea forecasts represent an average of the highest\\none-third of the combined wind wave and swell height.\\n\\n.TODAY...S wind 30 kt. Seas 15 ft.\\n.TONIGHT...SE wind 25 kt. Seas 13 ft. Rain.\\n.WED...SE wind 20 kt. Seas 11 ft.\\n.WED NIGHT...SE wind 15 kt. Seas 9 ft.\\n.THU...E wind 25 kt. Seas 7 ft.\\n.FRI...NW wind 15 kt. Seas 6 ft.\\n.SAT...NW wind 25 kt. Seas 6 ft.\",\n                \"instruction\": null,\n                \"response\": \"Avoid\",\n                \"parameters\": {\n                    \"AWIPSidentifier\": [\n                        \"CWFALU\"\n                    ],\n                    \"WMOidentifier\": [\n                        \"FZAK52 PAFC 021149\"\n                    ],\n                    \"NWSheadline\": [\n                        \"SMALL CRAFT ADVISORY THROUGH WEDNESDAY\"\n                    ],\n                    \"BLOCKCHANNEL\": [\n                        \"EAS\",\n                        \"NWEM\",\n                        \"CMAS\"\n                    ],\n                    \"VTEC\": [\n                        \"/O.NEW.PAFC.SC.Y.3139.251202T1100Z-251204T0200Z/\"\n                    ],\n                    \"eventEndingTime\": [\n                        \"2025-12-03T17:00:00-09:00\"\n                    ]\n                },\n                \"scope\": \"Public\",\n                \"code\": \"IPAWSv1.0\",\n                \"language\": \"en-US\",\n                \"web\": \"http://www.weather.gov\",\n                \"eventCode\": {\n                    \"SAME\": [\n                        \"NWS\"\n                    ],\n                    \"NationalWeatherService\": [\n                        \"SCY\"\n                    ]\n                }\n            }\n        },\n        {\n            \"id\": \"https://api.weather.gov/alerts/urn:oid:2.49.0.1.840.0.8d8456a64db8f93a127de0b73ddc98c3f937e864.025.1\",\n            \"type\": \"Feature\",\n            \"geometry\": null,\n            \"properties\": {\n                \"@id\": \"https://api.weather.gov/alerts/urn:oid:2.49.0.1.840.0.8d8456a64db8f93a127de0b73ddc98c3f937e864.025.1\",\n                \"@type\": \"wx:Alert\",\n                \"id\": \"urn:oid:2.49.0.1.840.0.8d8456a64db8f93a127de0b73ddc98c3f937e864.025.1\",\n                \"areaDesc\": \"Adak to Kiska Bering Side\",\n                \"geocode\": {\n                    \"SAME\": [\n                        \"058784\"\n                    ],\n                    \"UGC\": [\n                        \"PKZ784\"\n                    ]\n                },\n                \"affectedZones\": [\n                    \"https://api.weather.gov/zones/forecast/PKZ784\"\n                ],\n                \"references\": [],\n                \"sent\": \"2025-12-02T02:49:00-09:00\",\n                \"effective\": \"2025-12-02T02:49:00-09:00\",\n                \"onset\": \"2025-12-02T02:00:00-09:00\",\n                \"expires\": \"2025-12-02T15:45:00-09:00\",\n                \"ends\": \"2025-12-03T17:00:00-09:00\",\n                \"status\": \"Actual\",\n                \"messageType\": \"Alert\",\n                \"category\": \"Met\",\n                \"severity\": \"Moderate\",\n                \"certainty\": \"Likely\",\n                \"urgency\": \"Expected\",\n                \"event\": \"Gale Warning\",\n                \"sender\": \"w-nws.webmaster@noaa.gov\",\n                \"senderName\": \"NWS Anchorage AK\",\n                \"headline\": \"Gale Warning issued December 2 at 2:49AM AKST until December 3 at 5:00PM AKST by NWS Anchorage AK\",\n                \"description\": \"Coastal Waters Forecast for Southwest Alaska+Bristol Bay+The\\nAlaska Peninsula Waters and the Aleutian Islands up to 100 nm out.\\n\\nWind forecasts reflect the predominant speed and direction\\nexpected. Sea forecasts represent an average of the highest\\none-third of the combined wind wave and swell height.\\n\\n.TODAY...N wind 45 kt. Seas 29 ft. Rain.\\n.TONIGHT...N wind 40 kt. Seas 28 ft. Rain.\\n.WED...N wind 40 kt diminishing to 30 kt in the afternoon. Seas\\n28 ft.\\n.WED NIGHT...NE wind 30 kt. Seas 20 ft.\\n.THU...E wind 30 kt. Seas 15 ft.\\n.FRI...W wind 20 kt. Seas 12 ft.\\n.SAT...E wind 15 kt. Seas 11 ft.\",\n                \"instruction\": null,\n                \"response\": \"Avoid\",\n                \"parameters\": {\n                    \"AWIPSidentifier\": [\n                        \"CWFALU\"\n                    ],\n                    \"WMOidentifier\": [\n                        \"FZAK52 PAFC 021149\"\n                    ],\n                    \"NWSheadline\": [\n                        \"GALE WARNING THROUGH WEDNESDAY\"\n                    ],\n                    \"BLOCKCHANNEL\": [\n                        \"EAS\",\n                        \"NWEM\",\n                        \"CMAS\"\n                    ],\n                    \"VTEC\": [\n                        \"/O.NEW.PAFC.GL.W.3162.251202T1100Z-251204T0200Z/\"\n                    ],\n                    \"eventEndingTime\": [\n                        \"2025-12-03T17:00:00-09:00\"\n                    ]\n                },\n                \"scope\": \"Public\",\n                \"code\": \"IPAWSv1.0\",\n                \"language\": \"en-US\",\n                \"web\": \"http://www.weather.gov\",\n                \"eventCode\": {\n                    \"SAME\": [\n                        \"NWS\"\n                    ],\n                    \"NationalWeatherService\": [\n                        \"GLW\"\n                    ]\n                }\n            }\n        },\n        {\n            \"id\": \"https://api.weather.gov/alerts/urn:oid:2.49.0.1.840.0.8d8456a64db8f93a127de0b73ddc98c3f937e864.026.1\",\n            \"type\": \"Feature\",\n            \"geometry\": null,\n            \"properties\": {\n                \"@id\": \"https://api.weather.gov/alerts/urn:oid:2.49.0.1.840.0.8d8456a64db8f93a127de0b73ddc98c3f937e864.026.1\",\n                \"@type\": \"wx:Alert\",\n                \"id\": \"urn:oid:2.49.0.1.840.0.8d8456a64db8f93a127de0b73ddc98c3f937e864.026.1\",\n                \"areaDesc\": \"Adak to Kiska Pacific Side\",\n                \"geocode\": {\n                    \"SAME\": [\n                        \"058785\"\n                    ],\n                    \"UGC\": [\n                        \"PKZ785\"\n                    ]\n                },\n                \"affectedZones\": [\n                    \"https://api.weather.gov/zones/forecast/PKZ785\"\n                ],\n                \"references\": [],\n                \"sent\": \"2025-12-02T02:49:00-09:00\",\n                \"effective\": \"2025-12-02T02:49:00-09:00\",\n                \"onset\": \"2025-12-02T02:00:00-09:00\",\n                \"expires\": \"2025-12-02T15:45:00-09:00\",\n                \"ends\": \"2025-12-03T17:00:00-09:00\",\n                \"status\": \"Actual\",\n                \"messageType\": \"Alert\",\n                \"category\": \"Met\",\n                \"severity\": \"Moderate\",\n                \"certainty\": \"Likely\",\n                \"urgency\": \"Expected\",\n                \"event\": \"Gale Warning\",\n                \"sender\": \"w-nws.webmaster@noaa.gov\",\n                \"senderName\": \"NWS Anchorage AK\",\n                \"headline\": \"Gale Warning issued December 2 at 2:49AM AKST until December 3 at 5:00PM AKST by NWS Anchorage AK\",\n                \"description\": \"Coastal Waters Forecast for Southwest Alaska+Bristol Bay+The\\nAlaska Peninsula Waters and the Aleutian Islands up to 100 nm out.\\n\\nWind forecasts reflect the predominant speed and direction\\nexpected. Sea forecasts represent an average of the highest\\none-third of the combined wind wave and swell height.\\n\\n.TODAY...N wind 45 kt. Seas 24 ft.\\n.TONIGHT...N wind 40 kt. Seas 21 ft.\\n.WED...N wind 35 kt. Seas 20 ft.\\n.WED NIGHT...N wind 30 kt. Seas 15 ft.\\n.THU...E wind 30 kt. Seas 10 ft.\\n.FRI...W wind 25 kt. Seas 16 ft.\\n.SAT...E wind 15 kt. Seas 15 ft.\",\n                \"instruction\": null,\n                \"response\": \"Avoid\",\n                \"parameters\": {\n                    \"AWIPSidentifier\": [\n                        \"CWFALU\"\n                    ],\n                    \"WMOidentifier\": [\n                        \"FZAK52 PAFC 021149\"\n                    ],\n                    \"NWSheadline\": [\n                        \"GALE WARNING THROUGH WEDNESDAY\"\n                    ],\n                    \"BLOCKCHANNEL\": [\n                        \"EAS\",\n                        \"NWEM\",\n                        \"CMAS\"\n                    ],\n                    \"VTEC\": [\n                        \"/O.NEW.PAFC.GL.W.3163.251202T1100Z-251204T0200Z/\"\n                    ],\n                    \"eventEndingTime\": [\n                        \"2025-12-03T17:00:00-09:00\"\n                    ]\n                },\n                \"scope\": \"Public\",\n                \"code\": \"IPAWSv1.0\",\n                \"language\": \"en-US\",\n                \"web\": \"http://www.weather.gov\",\n                \"eventCode\": {\n                    \"SAME\": [\n                        \"NWS\"\n                    ],\n                    \"NationalWeatherService\": [\n                        \"GLW\"\n                    ]\n                }\n            }\n        },\n        {\n            \"id\": \"https://api.weather.gov/alerts/urn:oid:2.49.0.1.840.0.8d8456a64db8f93a127de0b73ddc98c3f937e864.021.1\",\n            \"type\": \"Feature\",\n            \"geometry\": null,\n            \"properties\": {\n                \"@id\": \"https://api.weather.gov/alerts/urn:oid:2.49.0.1.840.0.8d8456a64db8f93a127de0b73ddc98c3f937e864.021.1\",\n                \"@type\": \"wx:Alert\",\n                \"id\": \"urn:oid:2.49.0.1.840.0.8d8456a64db8f93a127de0b73ddc98c3f937e864.021.1\",\n                \"areaDesc\": \"Seguam to Adak Bering Side out to 15 NM\",\n                \"geocode\": {\n                    \"SAME\": [\n                        \"058780\"\n                    ],\n                    \"UGC\": [\n                        \"PKZ780\"\n                    ]\n                },\n                \"affectedZones\": [\n                    \"https://api.weather.gov/zones/forecast/PKZ780\"\n                ],\n                \"references\": [],\n                \"sent\": \"2025-12-02T02:49:00-09:00\",\n                \"effective\": \"2025-12-02T02:49:00-09:00\",\n                \"onset\": \"2025-12-02T02:00:00-09:00\",\n                \"expires\": \"2025-12-02T15:45:00-09:00\",\n                \"ends\": \"2025-12-03T17:00:00-09:00\",\n                \"status\": \"Actual\",\n                \"messageType\": \"Alert\",\n                \"category\": \"Met\",\n                \"severity\": \"Moderate\",\n                \"certainty\": \"Likely\",\n                \"urgency\": \"Expected\",\n                \"event\": \"Gale Warning\",\n                \"sender\": \"w-nws.webmaster@noaa.gov\",\n                \"senderName\": \"NWS Anchorage AK\",\n                \"headline\": \"Gale Warning issued December 2 at 2:49AM AKST until December 3 at 5:00PM AKST by NWS Anchorage AK\",\n                \"description\": \"Coastal Waters Forecast for Southwest Alaska+Bristol Bay+The\\nAlaska Peninsula Waters and the Aleutian Islands up to 100 nm out.\\n\\nWind forecasts reflect the predominant speed and direction\\nexpected. Sea forecasts represent an average of the highest\\none-third of the combined wind wave and swell height.\\n\\n.TODAY...N wind 45 kt. Seas 29 ft. Rain and snow.\\n.TONIGHT...N wind 45 kt. Seas 29 ft. Rain and snow.\\n.WED...N wind 35 kt. Seas 27 ft. Rain.\\n.WED NIGHT...N wind 30 kt. Seas 22 ft.\\n.THU...NE wind 30 kt. Seas 16 ft.\\n.FRI...N wind 15 kt. Seas 8 ft.\\n.SAT...NE wind 15 kt. Seas 7 ft.\",\n                \"instruction\": null,\n                \"response\": \"Avoid\",\n                \"parameters\": {\n                    \"AWIPSidentifier\": [\n                        \"CWFALU\"\n                    ],\n                    \"WMOidentifier\": [\n                        \"FZAK52 PAFC 021149\"\n                    ],\n                    \"NWSheadline\": [\n                        \"GALE WARNING THROUGH WEDNESDAY\"\n                    ],\n                    \"BLOCKCHANNEL\": [\n                        \"EAS\",\n                        \"NWEM\",\n                        \"CMAS\"\n                    ],\n                    \"VTEC\": [\n                        \"/O.NEW.PAFC.GL.W.3158.251202T1100Z-251204T0200Z/\"\n                    ],\n                    \"eventEndingTime\": [\n                        \"2025-12-03T17:00:00-09:00\"\n                    ]\n                },\n                \"scope\": \"Public\",\n                \"code\": \"IPAWSv1.0\",\n                \"language\": \"en-US\",\n                \"web\": \"http://www.weather.gov\",\n                \"eventCode\": {\n                    \"SAME\": [\n                        \"NWS\"\n                    ],\n                    \"NationalWeatherService\": [\n                        \"GLW\"\n                    ]\n                }\n            }\n        }\n    ],\n    \"title\": \"Current watches, warnings, and advisories\",\n    \"updated\": \"2025-12-03T16:14:55+00:00\"\n}" -> [w10 _]
    frame False {
    }
    frame True {
      n2 = call <vilib>:"GET.vi"("url"="https://api.weather.gov/alerts/active") -> ("body"=w11:string)  [unwired: 11 in, 3 out]
    }
  }
  n3 = call "Config From JSON.vi"("JSON"=w7) -> ("error out"=w3:errorcluster, "Config"=w6:refnum<class "Config Manager.lvclass">)  [unwired: 9 in]
  n4 = control-ref of="Tree"() -> (w4:refnum<vi>)
  n5 = call "Root Element.vi"("error in (no error)"=w3, "Config Manager in"=w6) -> ("error out"=w2:errorcluster, "Root Element"=w5:refnum<class "Config Element.lvclass">)  [unwired: 7 in, 1 out]
  n6 = call "Populate Tree View.vi"("Tree"=w4, "error in (no error)"=w2, "Element"=w5) -> ("error out"=→"error out":errorcluster)  [unwired: 8 in]
